vi "BasicFPGATest.vi"() -> ()   [LabVIEW 2015]
uses:
  <vilib>/Platform/TimedLoop/XDataNode/timing_clust.ctl
  <vilib>/Platform/TimedLoop/XDataNode/nitl_modes.ctl
  <vilib>/Platform/TimedLoop/XDataNode/wakeup.ctl
  <vilib>/rvi/Emulation/niFpgaGetClockAttributes.vi
  <vilib>/rvi/Emulation/niFpgaSctlEmulationGetInTimedLoop.vi
  <vilib>/rvi/Emulation/niFpgaEmulationReportErrorSimple.vi
  TickTocks/Tock1.vi
  <vilib>/rvi/Emulation/niFpgaCriticalErrorInLSC.vi
  TickTocks/Tick1.vi
  TickTocks/Tick0.vi
  TickTocks/Tock0.vi
  TickTocks/Tock2.vi
  TickTocks/Tick2.vi
  <vilib>/Platform/TimedLoop/XDataNode/XDataNode.xnode
  <vilib>/Platform/TimedLoop/XDataNode/XDNodeRunTimeDep.lvlib
  Timers.lvlib
panel:
  in  "resetMaxTime":bool
  out "MaxTimes":u32[](array[numeric])
  in  "SCTL_ticks":u16
  out "tock overhead":u32
  out "tick overhead":u32
  out "loop time":u32
  in  "delay":u32 caption="Delay"
  out "Times":u32[](array[numeric])
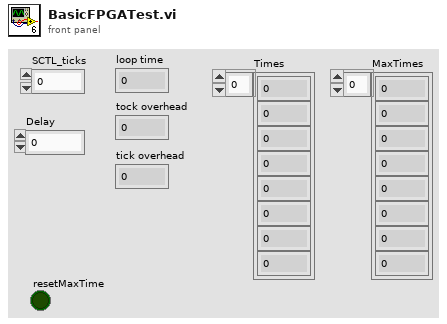
[diagram p1: front panel]
types:
  T1 = typedef "Timers.lvlib/TimerRegisters.ctl" = cluster{"Tick0":refnum<k21>, "Tock0":refnum<k21>, "Tick1":refnum<k21>, "Tock1":refnum<k21>, "Tick2":refnum<k21>, "Tock2":refnum<k21>, "Tick3":refnum<k21>, "Tock3":refnum<k21>, "Tick4":refnum<k21>, "Tock4":refnum<k21>, "Tick5":refnum<k21>, "Tock5":refnum<k21>, "Tick6":refnum<k21>, "Tock6":refnum<k21>, "Tick7":refnum<k21>, "Tock7":refnum<k21>}
  T2 = typedef "XDNodeRunTimeDep.lvlib/timing_clust.ctl" = cluster{"Expected End [f-1]":u64, "Actual End [f-1]":u64, "Finished Late? [f-1]":bool, "Expected End [i-1]":u64, "Actual End [i-1]":u64, "Finished Late? [i-1]":bool, "Expected Start [i]":u64, "Actual Start [i]":u64, "Expected Start [f]":u64, "Actual Start [f]":u64, "Source Name":string, "Structure Name":string, "Period":i64, "Deadline":i64, "Offset":i64, "Start":i64, "Priority":i32, "Timeout":i32, "Mode":T3, "Wakeup Reason":T4, "Error":errorcluster, "Source Type":string, "Secondary Source Type":string, "Global End Time":u64, "Global Start Time":u64, "Frame Duration":u64, "Iteration Duration":u64, "Assigned CPU":i32, "I/O Scan Engine Mode":u32}
  T3 = typedef "XDNodeRunTimeDep.lvlib/nitl_modes.ctl" = enum32{"No Change", "Process missed periods, maintain original phase", "Discard missed periods, maintain original phase", "Process missed periods, ignore original phase", "Discard missed periods, ignore original phase"}
  T4 = typedef "XDNodeRunTimeDep.lvlib/wakeup.ctl" = enum32{"Normal", "Aborted", "Asynchronous wakeup", "Timing source error", "Timed loop error", "Timeout"}
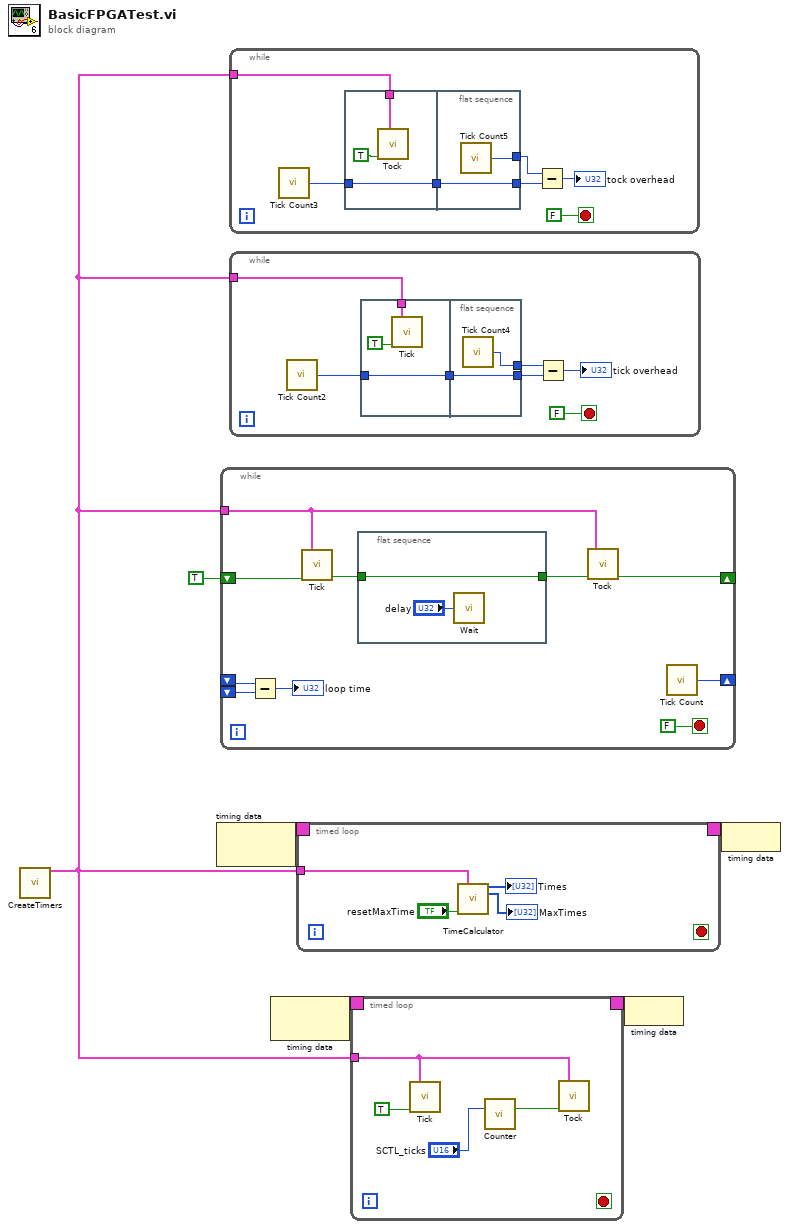
[diagram p0: block diagram]
diagram:
  n1 = call "CreateTimers.vi"() -> ("TimerRegisters"=w2:T1)  [unwired: 15 in]
  n2 = node-c288() -> (w6:T2)  [unwired: 1 in]
  n3 = while {
    tunnel: w2 -> [w9]
    shift-right: [w15] -> _
    shift-left: _ -> [w13]
    shift-left: _ -> [w14]
    shift-right: [w7] -> _
    shift-left: TRUE ("valid input") -> [w8]
    stop <- FALSE stop-if-true
    n4 = Subtract(x=w13, y=w14) -> (x-y=→"loop time":u32)
    n5 = call-poly "Tick.vi"("TimerRegisters"=w9, "valid input"=w8) -> ("valid output"=w11:bool)  [unwired: 13 in]
    n6 = flat-sequence {
      tunnel: [w17] -> w10
      tunnel: w11 -> [w17]
      frame #0 {
        n7 = call "Wait"("Count(Ticks)"="delay") -> ()  [unwired: 1 out]
      }
    }
    n8 = call-poly "Tock.vi"("TimerRegisters"=w9, "valid input"=w10) -> ("valid output"=w7:bool)  [unwired: 13 in]
    n9 = call "Tick Count"() -> ("Tick Count(Ticks)"=w15:u32)
  }
  n10 = while {
    tunnel: w2 -> [w24]
    stop <- FALSE stop-if-true
    n11 = call "Tick Count3"() -> ("Tick Count(Ticks)"=w23:u32)
    n12 = flat-sequence {
      tunnel: w24 -> [w27]
      tunnel: w23 -> [w28]
      tunnel: [w28] -> w21
      tunnel: [w30] -> w22
      tunnel: w21 -> [w29]
      tunnel: [w29] -> w20
      frame #0 {
        n13 = call-poly "Tock.vi"("TimerRegisters"=w27, "valid input"=TRUE) -> ()  [unwired: 13 in, 1 out]
      }
      frame #1 {
        n14 = call "Tick Count5"() -> ("Tick Count(Ticks)"=w30:u32)
      }
    }
    n15 = Subtract(x=w22, y=w20) -> (x-y=→"tock overhead":u32)
  }
  n16 = while {
    tunnel: w2 -> [w36]
    stop <- FALSE stop-if-true
    n17 = call "Tick Count2"() -> ("Tick Count(Ticks)"=w34:u32)
    n18 = flat-sequence {
      tunnel: w36 -> [w39]
      tunnel: w34 -> [w40]
      tunnel: [w40] -> w32
      tunnel: [w42] -> w33
      tunnel: w32 -> [w42]
      tunnel: [w41] -> w31
      frame #0 {
        n19 = call-poly "Tick.vi"("TimerRegisters"=w39, "valid input"=TRUE) -> ()  [unwired: 13 in, 1 out]
      }
      frame #1 {
        n20 = call "Tick Count4"() -> ("Tick Count(Ticks)"=w41:u32)
      }
    }
    n21 = Subtract(x=w31, y=w33) -> (x-y=→"tick overhead":u32)
  }
  n22 = node-c288() -> (w4:T2)  [unwired: 1 in]
  n23 = timed-loop {
    timing: w6 -> [_]
    timing-out: [_] -> w5
    tunnel: w2 -> [w45]
    stop <- _ stop-if-true
    n24 = call "TimeCalculator.vi"("TimerRegisters"=w45, "resetMaxTime"="resetMaxTime") -> ("Times"=→"Times":u32[], "MaxTimes"=→"MaxTimes":u32[])  [unwired: 12 in]
  }
  n25 = timed-loop {
    timing: w4 -> [_]
    timing-out: [_] -> w3
    tunnel: w2 -> [w50]
    stop <- _ stop-if-true
    n26 = call-poly "Tick.vi"("TimerRegisters"=w50, "valid input"=TRUE) -> ()  [unwired: 13 in, 1 out]
    n27 = call "Counter.vi"("ticks"="SCTL_ticks") -> ("ding"=w49:bool)  [unwired: 14 in]
    n28 = call-poly "Tock.vi"("TimerRegisters"=w50, "valid input"=w49) -> ()  [unwired: 13 in, 1 out]
  }
  n29 = node-c288(w3) -> ()
  n30 = node-c288(w5) -> ()
